vi "input tunnel.vi"() -> ()   [LabVIEW 2023]
panel:
  out "二维数组  concatenating":i32[][](array[numeric])
  out "last value":i32[](array[numeric])
  out "concatenating":i32[](array[numeric])
  out "indexing":i32[][](array[numeric])
  out "conditional indexing":i32[](array[numeric])
  out "last value":i32
  out "indexing":i32[](array[numeric])
  out "conditional indexing":i32[](array[numeric])
  # "数组输出通道"
  # "输入数 为一个实数的时候"
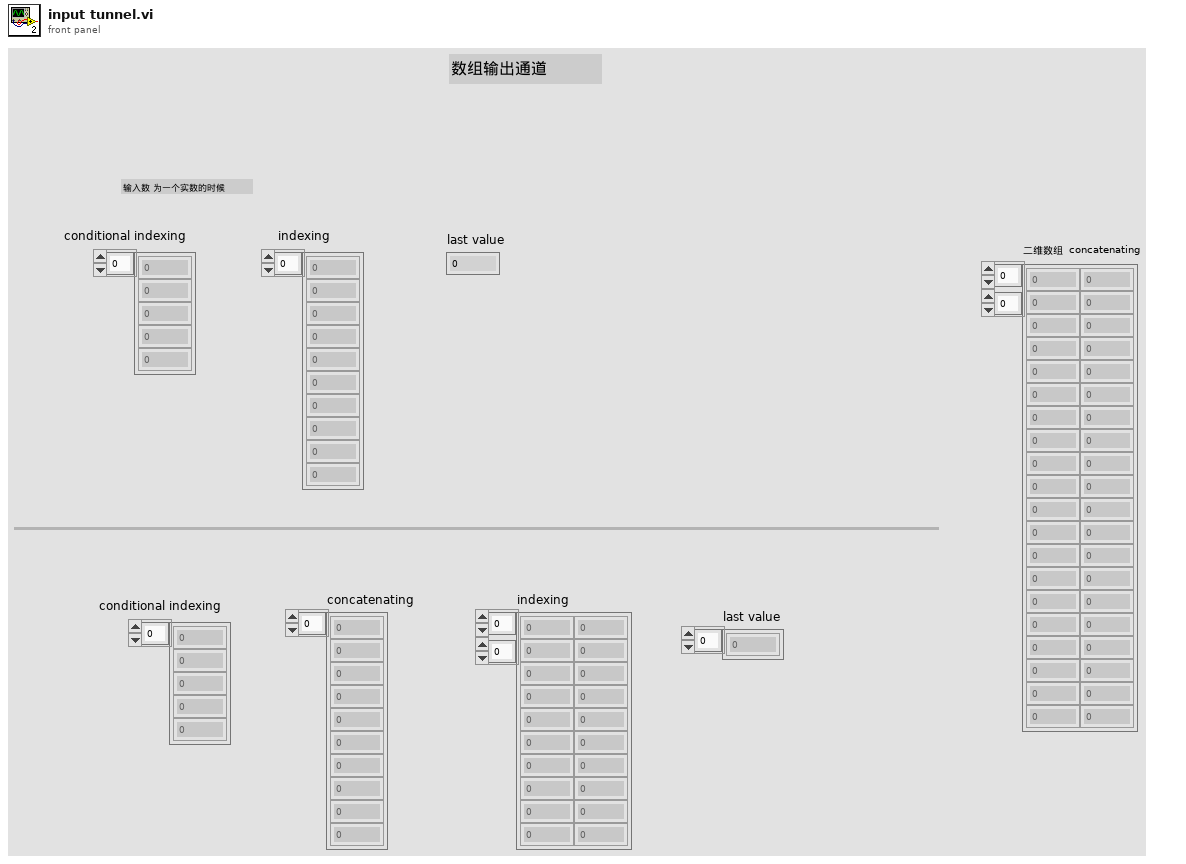
[diagram p1: front panel]
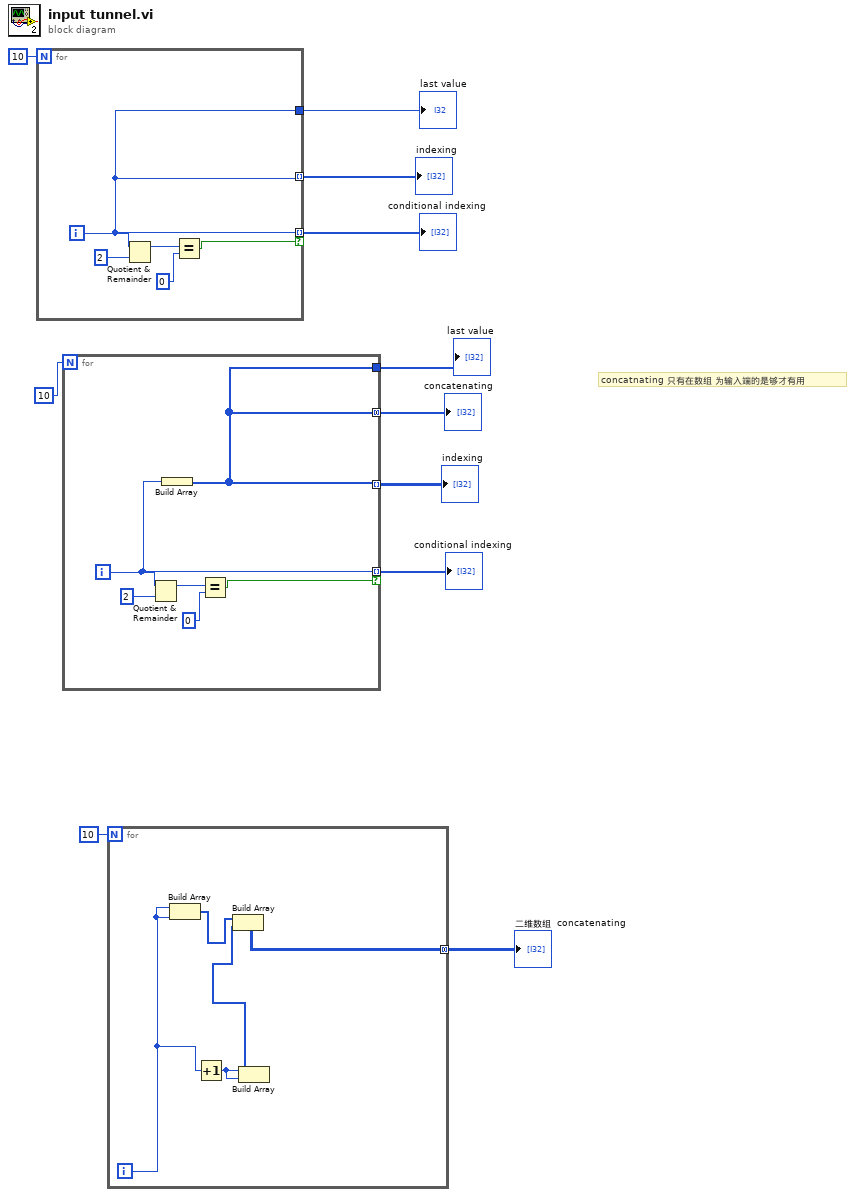
[diagram p0: block diagram]
diagram:
  # "concatnating 只有在数组 为输入端的是够才有用"
  n1 = for {
    N: 10 -> [_]
    tunnel: [w12] -> w10 mode=indexing if=w13
    tunnel: [w12] -> w9 mode=indexing
    tunnel: [w12] -> w8
    i -> [w12]
    n2 = Quotient & Remainder(x=w12, y=2) -> (x-y*floor(x/y)=w15:i32)  [unwired: 1 out]
    n3 = Equal?(x=w15, y=0) -> (x = y?=w13:bool)
  }
  "conditional indexing" <- w10
  "indexing" <- w9
  "last value" <- w8
  n4 = for {
    N: 10 -> [_]
    tunnel: [w18] -> w6 mode=indexing if=w19
    tunnel: [w17] -> w5 mode=indexing
    tunnel: [w17] -> w4 mode=concatenating
    tunnel: [w17] -> w3
    i -> [w18]
    n5 = Quotient & Remainder(x=w18, y=2) -> (x-y*floor(x/y)=w21:i32)  [unwired: 1 out]
    n6 = Build Array(w18) -> (w17:i32[])
    n7 = Equal?(x=w21, y=0) -> (x = y?=w19:bool)
  }
  "conditional indexing" <- w6
  "indexing" <- w5
  "concatenating" <- w4
  "last value" <- w3
  n8 = for {
    N: 10 -> [_]
    tunnel: [w25] -> w1 mode=concatenating
    i -> [w24]
    n9 = Build Array(w24, w24) -> (w27:i32[])
    n10 = Increment(x=w24) -> (x+1=w23:i32)
    n11 = Build Array(w23, w23) -> (w26:i32[])
    n12 = Build Array(w27, w26) -> (w25:i32[][])
  }
  "二维数组  concatenating" <- w1
